vi "Actor Core.vi"(8 "error in":errorcluster, 11 "Test-MM in":refnum<class "Test-MM.lvclass">) -> (0 "error out":errorcluster, 3 "Actor out":refnum<class "Actor.lvclass">)   [LabVIEW 2020, in "Test-MM.lvlib" / "Test-MM.lvclass"]
doc: "(<B>Filename</B>: Actor Framework.lvlib:Actor.lvclass:Actor Core.vi)\n\nReceives messages to the actor, reacts to them, and initiates any error handling that may shut the actor down.\n\nDescendant classes may override this VI to append parallel tasks for the actor to complete while it handles messages. Overrides use the Call Parent Class Method node."
uses:
  Test-MM.lvclass
  C:/Program Files (x86)/National Instruments/LabVIEW 2020/vi.lib/ActorFramework/Actor/Actor.lvclass
  <vilib>/ActorFramework/Actor/Actor.lvclass
  <vilib>/ActorFramework/Actor/Actor.lvclass/Actor.ctl
  <vilib>/ActorFramework/Message Enqueuer/Message Enqueuer.lvclass/Message Enqueuer.ctl
  <vilib>/ActorFramework/Message Enqueuer/Init from Existing Queue.vi
  <vilib>/ActorFramework/Message Enqueuer/Enqueue.vi
  Test-Client/Test-Client/Test-Client.lvclass
  <vilib>/ActorFramework/Stop Msg/Stop Msg.lvclass
  C:/Program Files (x86)/National Instruments/LabVIEW 2020/vi.lib/ActorFramework/Message/Message.lvclass
  <vilib>/ActorFramework/Message Priority Queue/Priority Enqueue.vi
  <vilib>/ActorFramework/Message Enqueuer/Message Enqueuer.lvclass
  MailboxManager/MailboxManager/MailboxManager.lvclass
  C:/Users/taylo/Projects/LabVIEW/ActorMailbox/MailboxManager/MailboxManager/MailboxManager.lvclass
  C:/Users/taylo/Projects/LabVIEW/ActorMailbox/MailboxClientInterface/MailboxClientInterface.lvclass
  C:/Users/taylo/Projects/LabVIEW/ActorMailbox/Example/Test-MM/Test-MM/Test-MM.lvclass
  ExternClient/MC-ExternClient/MC-ExternClient/MC-ExternClient.lvclass
  C:/Users/taylo/Projects/LabVIEW/ActorMailbox/MailboxClient/MailboxClient/MailboxClient.lvclass
  C:/Users/taylo/Projects/LabVIEW/ActorMailbox/Test-Client/Test-Client/Test-Client.lvclass
  C:/Users/taylo/Projects/LabVIEW/ActorMailbox/Example/ExternClient/MC-ExternClient/MC-ExternClient/MC-ExternClient.lvclass
panel:
  in  "Stop":bool
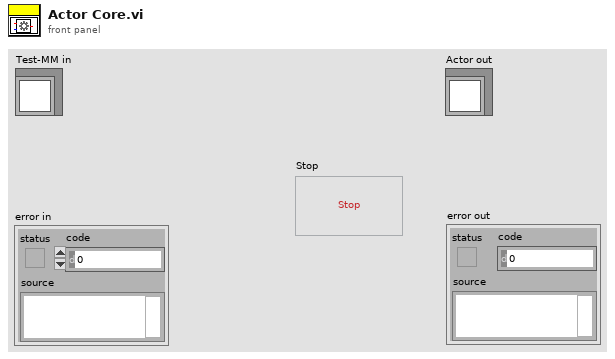
[diagram p1: front panel]
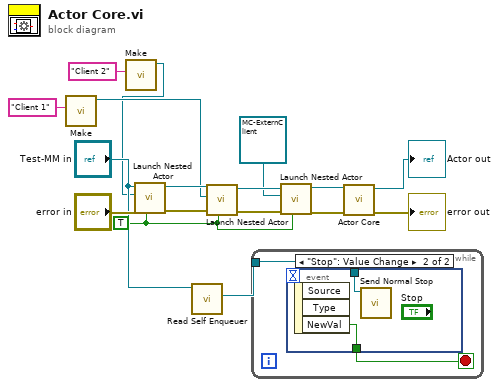
[diagram p0: block diagram]
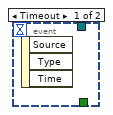
[diagram p2: hidden frame]
diagram:
  w4 = TRUE ("Open Actor Core front panel? (F)")
  n1 = call "Make.vi"("Actor"="Client 1") -> ("Test-Client out"=w10:refnum<class "Test-Client.lvclass">)  [unwired: 9 in, 1 out]
  n2 = call "Make.vi"("Actor"="Client 2") -> ("Test-Client out"=w7:refnum<class "Test-Client.lvclass">)  [unwired: 9 in, 1 out]
  n3 = call <vilib>:"Launch Nested Actor.vi"("Open Actor Core front panel? (F)"=w4, "error in (no error)"="error in", "Nested Actor"=w7, "Caller Actor in"="Test-MM in") -> ("error out"=w14:errorcluster, "Caller Actor out"=w13:refnum<class "Test-MM.lvclass">)  [unwired: 5 in, 1 out]
  n4 = call <vilib>:"Read Self Enqueuer.vi"("Actor"="Test-MM in") -> ("Self Enqueuer"=w11:refnum<class "Message Enqueuer.lvclass">)  [unwired: 10 in]
  n5 = call <vilib>:"Launch Nested Actor.vi"("Open Actor Core front panel? (F)"=w4, "error in (no error)"=w14, "Nested Actor"=w10, "Caller Actor in"=w13) -> ("error out"=w5:errorcluster, "Caller Actor out"=w6:refnum<class "Test-MM.lvclass">)  [unwired: 5 in, 1 out]
  n6 = while {
    tunnel: w11 -> [w19]
    stop <- w18 stop-if-true
    n7 = event shown="[1] \"Stop\": Value Change" {
      selector: _ -> [_ _]
      dyn-events: _ -> [_ _]
      timeout: _ -> [_ _]
      tunnel: w19 -> [_ w21]
      tunnel: [_ w20] -> w18
      event Timeout {
        n8 = event-data() -> ()  [unwired: 1 in, 3 out]
      }
      event "Stop": Value Change {
        n9 = event-data() -> ("NewVal"=w20:bool)  [unwired: 1 in, 2 out]
        n10 = call <vilib>:"Send Normal Stop.vi"("Message Enqueuer"=w21) -> ()  [unwired: 10 in, 1 out]
      }
    }
  }
  n11 = call <vilib>:"Launch Nested Actor.vi"("Open Actor Core front panel? (F)"=w4, "error in (no error)"=w5, "Nested Actor"=refnum<class "MC-ExternClient.lvclass"> refnum ("MC-ExternClient.lvlib:MC-ExternClient.lvclass"), "Caller Actor in"=w6) -> ("error out"=w2:errorcluster, "Caller Actor out"=w3:refnum<class "Test-MM.lvclass">)  [unwired: 5 in, 1 out]
  n12 = call-parent "Actor Core.vi"("error in"=w2, "Actor in"=w3) -> ("error out"=→"error out":errorcluster, "Actor out"=→"Actor out":refnum<class "Actor.lvclass">)  [unwired: 8 in]
